vi "Save Spectrogramme.vi"(8 "error in (no error)":errorcluster caption="entrée d'erreur (pas d'erreur)", 9 "sauvegarde":path, 10 "um":dbl, 11 "UI SA en entrée":refnum<class "UI SmarAct.lvclass">) -> (0 "error out":errorcluster caption="sortie d'erreur", 1 "file path saved":path, 3 "UI SA en sortie":refnum<class "UI SmarAct.lvclass">)   [LabVIEW 2024, in "UI SmarAct.lvclass"]
uses:
  UI SmarAct.lvclass
  UI SmarAct.lvclass/UI SmarAct.ctl
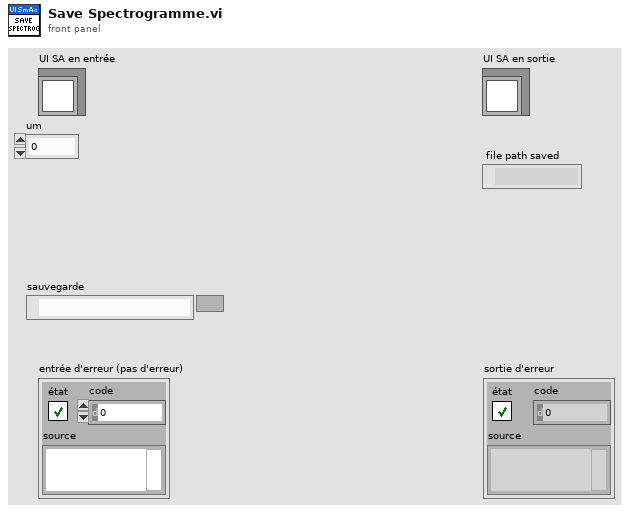
[diagram p1: front panel]
types:
  T1 = enum16{"open", "open or create", "create or replace", "create"}
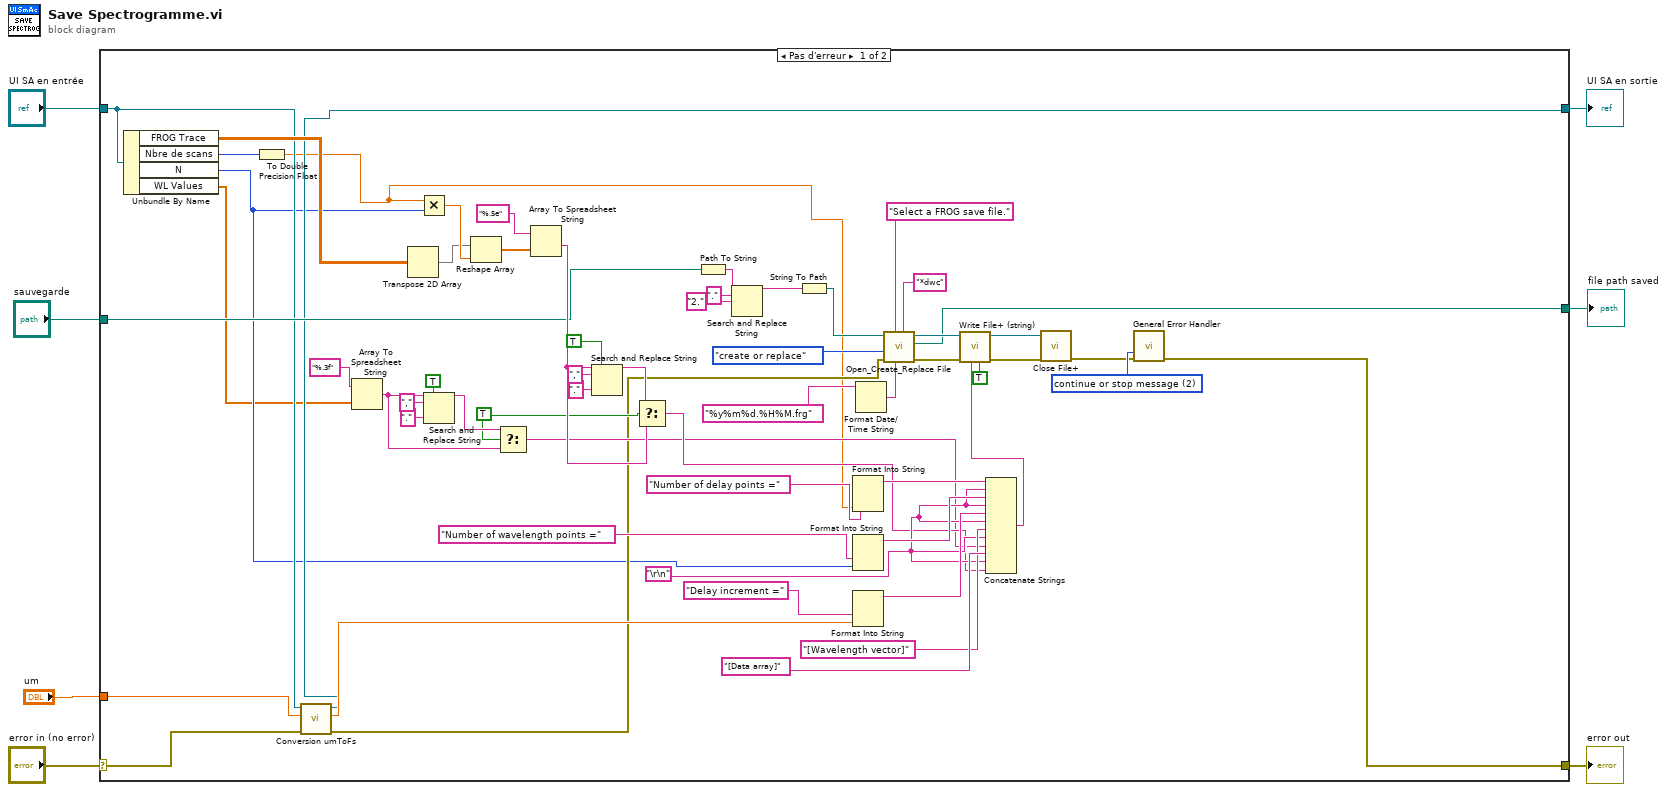
[diagram p0: block diagram]
diagram:
  n1 = case shown="Pas d'erreur" "error in (no error)" {
    selector: "error in (no error)" -> [w16 w69]
    tunnel: [w8 w69] -> w6
    tunnel: [w13 w68] -> w4
    tunnel: "UI SA en entrée" -> [w14 w68]
    tunnel: [w21 w67] -> w3
    tunnel: "sauvegarde" -> [w20 w67]
    tunnel: "um" -> [w17 _]
    frame No Error {
      w23 = TRUE ("s")
      w40 = "\r\n"
      w54 = u16 2 items=["no dialog", "OK message", "continue or stop message"] ("type of dialog (OK msg:1)")
      n2 = Unbundle By Name(w14) -> ("FROG Trace"=w19:dbl[][], "Nbre de scans"=w12:i32, "N"=w10:i32, "WL Values"=w9:dbl[])
      n3 = To Double Precision Float(number=w12) -> (double precision float=w11:dbl)
      n4 = call "Conversion umToFs.vi"("error in (no error)"=w16, "um"=w17, "UI SA en entrée"=w14) -> ("error out"=w15:errorcluster, "Fs"=w18:ext, "UI SA en sortie"=w13:refnum<class "UI SmarAct.lvclass">)  [unwired: 6 in]
      n5 = Array To Spreadsheet String(array=w9, 3:"%.3f" ("format (%.3f) 2")) -> (spreadsheet string=w22:string)  [unwired: 1 out]
      n6 = Transpose 2D Array(2D array=w19) -> (transposed array=w62:dbl[][])
      n7 = Multiply(x=w11, y=w10) -> (x*y=w64:dbl)
      n8 = Search and Replace String(replace all?=TRUE ("replace all? (F)"), input string=w22, search string=",", replace string="." ("replace string (\"\")")) -> (result string=w25:string)  [unwired: 4 in, 3 out]
      n9 = Reshape Array(w62, w64) -> (w63:dbl[])
      n10 = Select(t=w25, s=w23, f=w22) -> (s? t:f=w24:string)
      n11 = Array To Spreadsheet String(array=w63, 3:"%.5e" ("format (%.3f)")) -> (spreadsheet string=w30:string)  [unwired: 1 out]
      n12 = Search and Replace String(replace all?=TRUE ("replace all? (F)"), input string=w30, search string=",", replace string="." ("replace string (\"\")")) -> (result string=w31:string)  [unwired: 4 in, 3 out]
      n13 = Select(t=w31, s=w23, f=w30) -> (s? t:f=w29:string)
      n14 = Path To String(path=w20) -> (string=w39:string)
      n15 = Search and Replace String ("Rechercher et remplacer une chaîne")(input string=w39, search string="." ("chaîne recherchée"), replace string="2." ("chaîne de remplacement (\"\")")) -> (result string=w36:string)  [unwired: 5 in, 3 out]
      n16 = String To Path(string=w36) -> (path=w35:path)
      n17 = Format Into String("Number of delay points =" ("format (%.3f) 2"), w11) -> (resulting string=w47:string)  [unwired: 3 in, 1 out]
      n18 = Format Into String("Number of wavelength points =" ("format (%.3f) 2"), w10) -> (resulting string=w45:string)  [unwired: 3 in, 1 out]
      n19 = Format Into String("Delay increment =" ("format (%.3f) 2"), w18) -> (resulting string=w43:string)  [unwired: 3 in, 1 out]
      n20 = Format Date/Time String(time format string (%c)="%y%m%d.%H%M.frg") -> (date/time string=w60:string)  [unwired: 2 out]
      n21 = call <vilib>:"Open_Create_Replace File.vi"("pattern"="*dwc", "default name"=w60, "prompt"="Select a FROG save file.", "error in (no error)"=w15, "function (open:0)"=T1."create or replace", "file path"=w35) -> ("error out"=w50:errorcluster, "new file path"=w21:path, "refnum"=w53:refnum<file>)  [unwired: 1 in, 2 out]
      n22 = Concatenate Strings(w47, w40, w45, w40, w43, w40, "[Wavelength vector]" ("format (%.3f) 2"), w40, w24, "[Data array]" ("entrée 15"), w40, w29) -> (w48:string)
      n23 = call <vilib>:"Write File+ (string).vi"("convert eol? (no:F)"=TRUE, "string"=w48, "error in (no error)"=w50, "refnum"=w53) -> ("error out"=w49:errorcluster, "dup refnum"=w51:refnum<file>)  [unwired: 2 in, 2 out]
      n24 = call <vilib>:"Close File+.vi"("error in (no error)"=w49, "refnum"=w51) -> ("error out"=w52:errorcluster)  [unwired: 5 out]
      n25 = call <vilib>:"General Error Handler.vi"("type of dialog (OK msg:1)"=w54, "error in (no error)"=w52) -> ("error out"=w8:errorcluster)  [unwired: 1 in, 12 out]
    }
    frame Error {
    }
  }
  "error out" <- w6
  "UI SA en sortie" <- w4
  "file path saved" <- w3
